vi "Excel Set Cell Font.vi"(0 "report in":refnum<class "NI_report.lvclass">, 1 "auto format":i32(ring)=-4142 items=["xlRangeAutoFormat3DEffects1"=13, "xlRangeAutoFormat3DEffects2"=14, "xlRangeAutoFormatAccounting1"=4, "xlRangeAutoFormatAccounting2"=5, "xlRangeAutoFormatAccounting3"=6, "xlRangeAutoFormatAccounting4"=17, "xlRangeAutoFormatClassic1"=1, "xlRangeAutoFormatClassic2"=2, "xlRangeAutoFormatClassic3"=3, "xlRangeAutoFormatColor1"=7, "xlRangeAutoFormatColor2"=8, "xlRangeAutoFormatColor3"=9, "xlRangeAutoFormatList1"=10, "xlRangeAutoFormatList2"=11, "xlRangeAutoFormatList3"=12, "xlRangeAutoFormatLocalFormat1"=15, "xlRangeAutoFormatLocalFormat2"=16, "xlRangeAutoFormatLocalFormat3"=19, "xlRangeAutoFormatLocalFormat4"=20, "xlRangeAutoFormatReport1"=21, "xlRangeAutoFormatReport2"=22, "xlRangeAutoFormatReport3"=23, "xlRangeAutoFormatReport4"=24, "xlRangeAutoFormatReport5"=25, "xlRangeAutoFormatReport6"=26, "xlRangeAutoFormatReport7"=27, "xlRangeAutoFormatReport8"=28, "xlRangeAutoFormatReport9"=29, "xlRangeAutoFormatReport10"=30, "xlRangeAutoFormatClassicPivotTable"=31, "xlRangeAutoFormatTable1"=32, "xlRangeAutoFormatTable2"=33, "xlRangeAutoFormatTable3"=34, "xlRangeAutoFormatTable4"=35, "xlRangeAutoFormatTable5"=36, "xlRangeAutoFormatTable6"=37, "xlRangeAutoFormatTable7"=38, "xlRangeAutoFormatTable8"=39, "xlRangeAutoFormatTable9"=40, "xlRangeAutoFormatTable10"=41, "xlRangeAutoFormatPTNone"=42, "xlRangeAutoFormatNone"=-4142, "xlRangeAutoFormatSimple"=-4154], 5 "font":T1={"font name"="", "font size"=0.0, "bold"=0, "italic"=0, "underline"=0, "strike through"=0, "font color"=16777216} {"font size" format="%.2f"; "strike through" items=["Unchanged", "Yes", "No"]; "underline" items=["Unchanged", "Yes", "No"]; "italic" items=["Unchanged", "Yes", "No"]; "bold" items=["Unchanged", "Yes", "No"]}, 7 "start (-1, -1)":cluster{"row":i32, "column":i32}={"row"=-1, "column"=-1}, 9 "end (-1, -1)":cluster{"row":i32, "column":i32}={"row"=-1, "column"=-1}, 11 "error in (no error)":errorcluster, 12 "name (\"\")":string) -> (4 "report out":refnum<class "NI_report.lvclass">, 15 "error out":errorcluster)   [LabVIEW 2017, in "NI_Excel.lvclass"]
doc: "Sets the font of the cells specified by the <B>start</B> and <B>end</B> clusters or by a named range."
uses:
  <vilib>/Utility/NIReport.llb/Excel/NI_Excel.lvclass
  <vilib>/Utility/NIReport.llb/NI_report.lvclass
  <vilib>/addons/_office/_exclsub.llb/font.ctl
  C:/Program Files (x86)/National Instruments/LabVIEW 2017/vi.lib/Utility/NIReport.llb/NI_report.lvclass
  <vilib>/Utility/NIReport.llb/Excel/NI_Excel.lvclass/NI_Excel.ctl
  <vilib>/addons/_office/NI_ReportGenerationToolkit.lvlib
  <vilib>/Utility/NIReport.llb/NI_ReportGenerationCore.lvlib
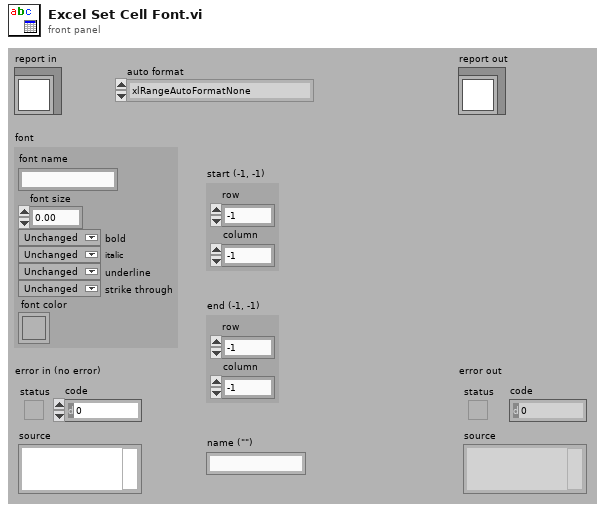
[diagram p1: front panel]
types:
  T1 = typedef "NI_ReportGenerationToolkit.lvlib/font.ctl" = cluster{"font name":string, "font size":dbl, "bold":u16, "italic":u16, "underline":u16, "strike through":u16, "font color":u32}
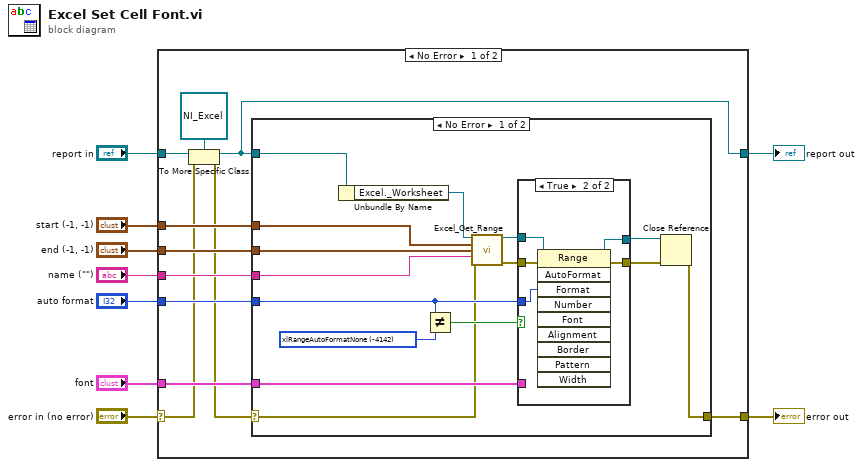
[diagram p0: block diagram]
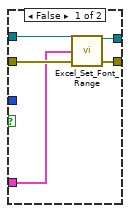
[diagram p2: hidden frame]
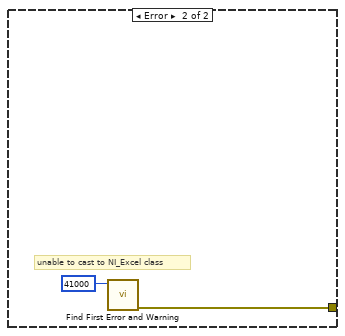
[diagram p3: hidden frame]
diagram:
  n1 = case shown="No Error" "error in (no error)" {
    selector: "error in (no error)" -> [w10 w49]
    tunnel: [w15 w49] -> w8
    tunnel: [w12 w48] -> w6
    tunnel: "report in" -> [w13 w48]
    tunnel: "start (-1, -1)" -> [w20 _]
    tunnel: "end (-1, -1)" -> [w19 _]
    tunnel: "auto format" -> [w18 _]
    tunnel: "name (\"\")" -> [w17 _]
    tunnel: "font" -> [w16 _]
    frame No Error {
      n2 = To More Specific Class(target class=refnum<class "NI_Excel.lvclass"> refnum ("report in"), reference=w13, error in=w10) -> (specific class reference=w12:refnum<class "NI_Excel.lvclass">, error out=w11:errorcluster)
      n3 = case shown="No Error" w11 {
        selector: w11 -> [w21 _]
        tunnel: w20 -> [w28 _]
        tunnel: w19 -> [w27 _]
        tunnel: w18 -> [w26 _]
        tunnel: w17 -> [w25 _]
        tunnel: w16 -> [w24 _]
        tunnel: [w23 w46] -> w15
        tunnel: w12 -> [w22 _]
        frame No Error {
          w33 = -4142 items=["xlRangeAutoFormat3DEffects1"=13, "xlRangeAutoFormat3DEffects2"=14, "xlRangeAutoFormatAccounting1"=4, "xlRangeAutoFormatAccounting2"=5, "xlRangeAutoFormatAccounting3"=6, "xlRangeAutoFormatAccounting4"=17, "xlRangeAutoFormatClassic1"=1, "xlRangeAutoFormatClassic2"=2, "xlRangeAutoFormatClassic3"=3, "xlRangeAutoFormatColor1"=7, "xlRangeAutoFormatColor2"=8, "xlRangeAutoFormatColor3"=9, "xlRangeAutoFormatList1"=10, "xlRangeAutoFormatList2"=11, "xlRangeAutoFormatList3"=12, "xlRangeAutoFormatLocalFormat1"=15, "xlRangeAutoFormatLocalFormat2"=16, "xlRangeAutoFormatLocalFormat3"=19, "xlRangeAutoFormatLocalFormat4"=20, "xlRangeAutoFormatReport1"=21, "xlRangeAutoFormatReport2"=22, "xlRangeAutoFormatReport3"=23, "xlRangeAutoFormatReport4"=24, "xlRangeAutoFormatReport5"=25, "xlRangeAutoFormatReport6"=26, "xlRangeAutoFormatReport7"=27, "xlRangeAutoFormatReport8"=28, "xlRangeAutoFormatReport9"=29, "xlRangeAutoFormatReport10"=30, "xlRangeAutoFormatClassicPivotTable"=31, "xlRangeAutoFormatTable1"=32, "xlRangeAutoFormatTable2"=33, "xlRangeAutoFormatTable3"=34, "xlRangeAutoFormatTable4"=35, "xlRangeAutoFormatTable5"=36, "xlRangeAutoFormatTable6"=37, "xlRangeAutoFormatTable7"=38, "xlRangeAutoFormatTable8"=39, "xlRangeAutoFormatTable9"=40, "xlRangeAutoFormatTable10"=41, "xlRangeAutoFormatPTNone"=42, "xlRangeAutoFormatNone"=-4142, "xlRangeAutoFormatSimple"=-4154] ("Format")
          n4 = Unbundle By Name(w22) -> ("Excel._Worksheet"=w29:refnum<k7>)
          n5 = Not Equal?(x=w26, y=w33) -> (x != y?=w32:bool)
          n6 = call <vilib>:"Excel_Get_Range.vi"("Excel._Worksheet"=w29, "start"=w28, "end"=w27, "name"=w25, "error in (no error)"=w21) -> ("Range"=w30:refnum<k7>, "error out"=w31:errorcluster)  [unwired: 5 in, 4 out]
          n7 = case shown="True" w32 {
            tunnel: w30 -> [w40 w45]
            tunnel: w31 -> [w39 w44]
            tunnel: w26 -> [_ w43]
            tunnel: [w38 w42] -> w34
            tunnel: [w37 w41] -> w35
            tunnel: w24 -> [w36 _]
            frame False {
              n8 = call <vilib>:"Excel_Set_Font_Range.vi"("Excel.Range"=w40, "font"=w36, "error in (no error)"=w39) -> ("Excel.Range out"=w37:refnum<k7>, "error out"=w38:errorcluster)  [unwired: 5 out]
            }
            frame True {
              n9 = invoke class="Range" method="AutoFormat"(reference=w45, error in=w44, "Format"=w43) -> (reference out=w41:refnum<k7>, error out=w42:errorcluster)  [unwired: 7 in, 8 out]
            }
          }
          n10 = Close Reference(reference=w35, error in (no error)=w34) -> (error out=w23:errorcluster)
        }
        frame Error {
          # "unable to cast to NI_Excel class"
          n11 = call <vilib>:"Find First Error and Warning.vi"("error code"=41000) -> ("error out"=w46:errorcluster)  [unwired: 2 in, 4 out]
        }
      }
    }
    frame Error {
    }
  }
  "error out" <- w8
  "report out" <- w6
